vi "di_oneshot_lite.vi"() -> ()   [LabVIEW 2020]
uses:
  <vilib>/Waveform/DWDTOps.llb/DWDT Analog to Digital.vi
panel:
  out "error out":errorcluster caption="错误输出"
  out "数字波形图":digitalwaveform(graph)
  in  "DiOneShotPoints":u32=1000
  in  "SamplePeriod":u32=10000 caption="SamplePeriod (ns)"
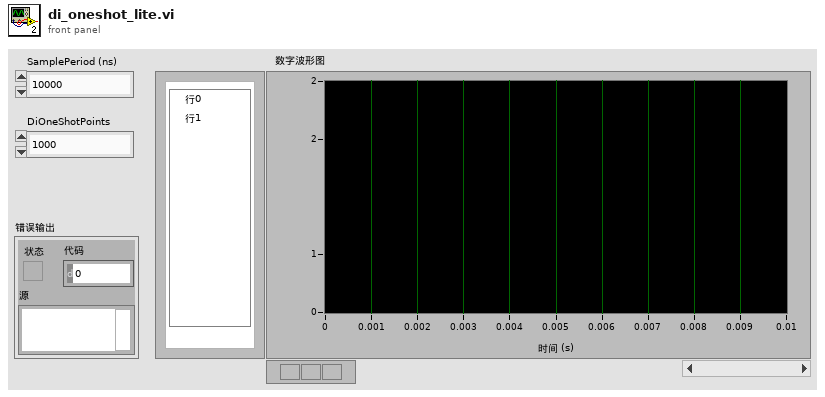
[diagram p1: front panel]
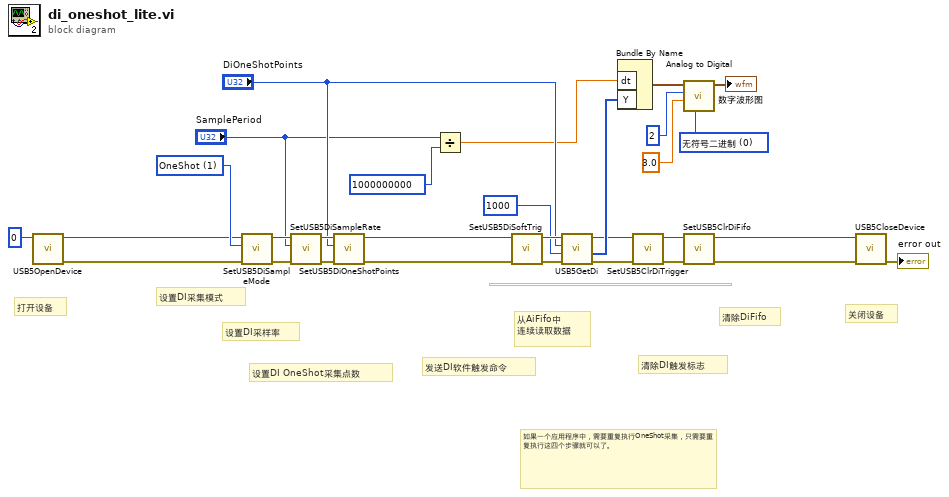
[diagram p0: block diagram]
diagram:
  w13 = u16 0 items=["无符号二进制", "二进制偏移量", "二进制补码"] ("data format (offset binary)")
  w29 = u8 1 items=["Continuous", "OneShot"] ("DiSampleMode")
  # "设置DI OneShot采集点数"
  # "设置DI采样率"
  # "设置DI采集模式"
  # "打开设备"
  # "从AiFifo中\n连续读取数据"
  # "发送DI软件触发命令"
  # "如果一个应用程序中，需要重复执行OneShot采集，只需要重复执行这四个步骤就可以了。"
  # "关闭设备"
  # "清除DiFifo"
  # "清除DI触发标志"
  n1 = call "USB5OpenDevice.vi"("DevIndex"=0) -> ("error out"=w2:errorcluster, "DevIndex Out"=w3:i32)  [unwired: 9 in]
  n2 = call "SetUSB5DiSampleMode.vi"("错误输入（无错误）"=w2, "DiSampleMode"=w29, "DevIndex"=w3) -> ("错误输出"=w28:errorcluster, "DevIndex Out"=w27:i32)  [unwired: 7 in]
  n3 = call "SetUSB5DiSampleRate.vi"("错误输入（无错误）"=w28, "SamplePeriod(ns)"="SamplePeriod", "DevIndex"=w27) -> ("错误输出"=w26:errorcluster, "DevIndex Out"=w25:i32)  [unwired: 7 in]
  n4 = call "SetUSB5DiOneShotPoints.vi"("错误输入（无错误）"=w26, "DiOneShotPoints"="DiOneShotPoints", "DevIndex"=w25) -> ("错误输出"=w24:errorcluster, "DevIndex Out"=w23:i32)  [unwired: 7 in]
  n5 = Divide(x="SamplePeriod", y=u32 1000000000) -> (x/y=w10:dbl)
  n6 = call "SetUSB5DiSoftTrig.vi"("错误输入（无错误）"=w24, "DevIndex"=w23) -> ("错误输出"=w21:errorcluster, "DevIndex Out"=w22:i32)  [unwired: 8 in]
  n7 = call "USB5GetDi.vi"("错误输入（无错误）"=w21, "TimeOut"=1000, "Points"="DiOneShotPoints", "DevIndex"=w22) -> ("错误输出"=w5:errorcluster, "Di"=w9:u8[], "DevIndex Out"=w6:i32)  [unwired: 4 in, 1 out]
  n8 = Bundle By Name("dt"=w10, "Y"=w9) -> (w12:waveform(u8))  [unwired: 1 in]
  n9 = call "SetUSB5ClrDiTrigger.vi"("错误输入（无错误）"=w5, "DevIndex"=w6) -> ("错误输出"=w8:errorcluster, "DevIndex Out"=w7:i32)  [unwired: 8 in]
  n10 = call-poly <vilib>:"Analog to Digital.vi"("data format (offset binary)"=w13, "full-scale range (pk-pk)"=3.0, "resolution (16 bit)"=2, "analog waveform"=w12) -> ("digital waveform"=→"数字波形图":digitalwaveform)  [unwired: 4 in, 3 out]
  n11 = call "SetUSB5ClrDiFifo.vi"("错误输入（无错误）"=w8, "DevIndex"=w7) -> ("错误输出"=w16:errorcluster, "DevIndex Out"=w17:i32)  [unwired: 8 in]
  n12 = call "USB5CloseDevice.vi"("错误输入（无错误）"=w16, "DevIndex"=w17) -> ("error out"=→"error out":errorcluster)  [unwired: 8 in, 1 out]
